vi "Struct Parse Variable Type.vi"(8 "error in":errorcluster, 11 "variant in":variant) -> (0 "error out":errorcluster, 1 "array dims":i16, 2 "data type":T1=enum."Real", 3 "type id":i16)   [LabVIEW 2013, in "GOLPI library.lvlib"]
doc: "Parses 'variable' data type. Obtains data types of the variable, array dimensions count."
uses:
  GOLPI library.lvlib
  Struct Data Types.ctl
panel:
  out "type string":i16[](array[numeric]) format="%04x"
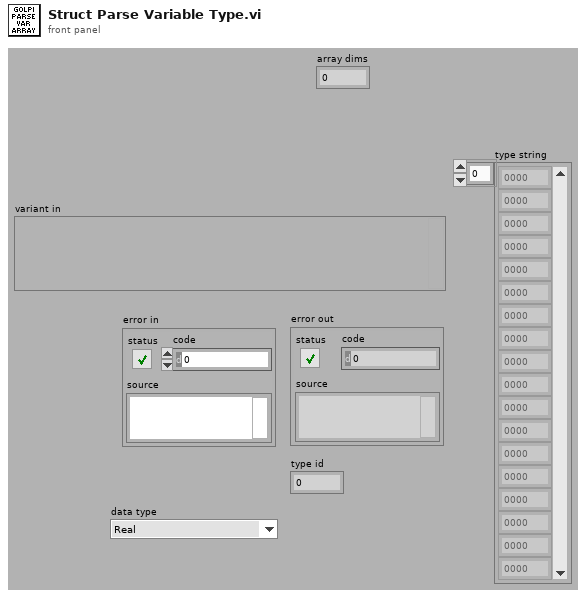
[diagram p1: front panel]
types:
  T1 = typedef "GOLPI library.lvlib/Struct Data Types.ctl" = enum16{"n/a", "Real", "Complex", "String/path", "Cluster", "Bool"}
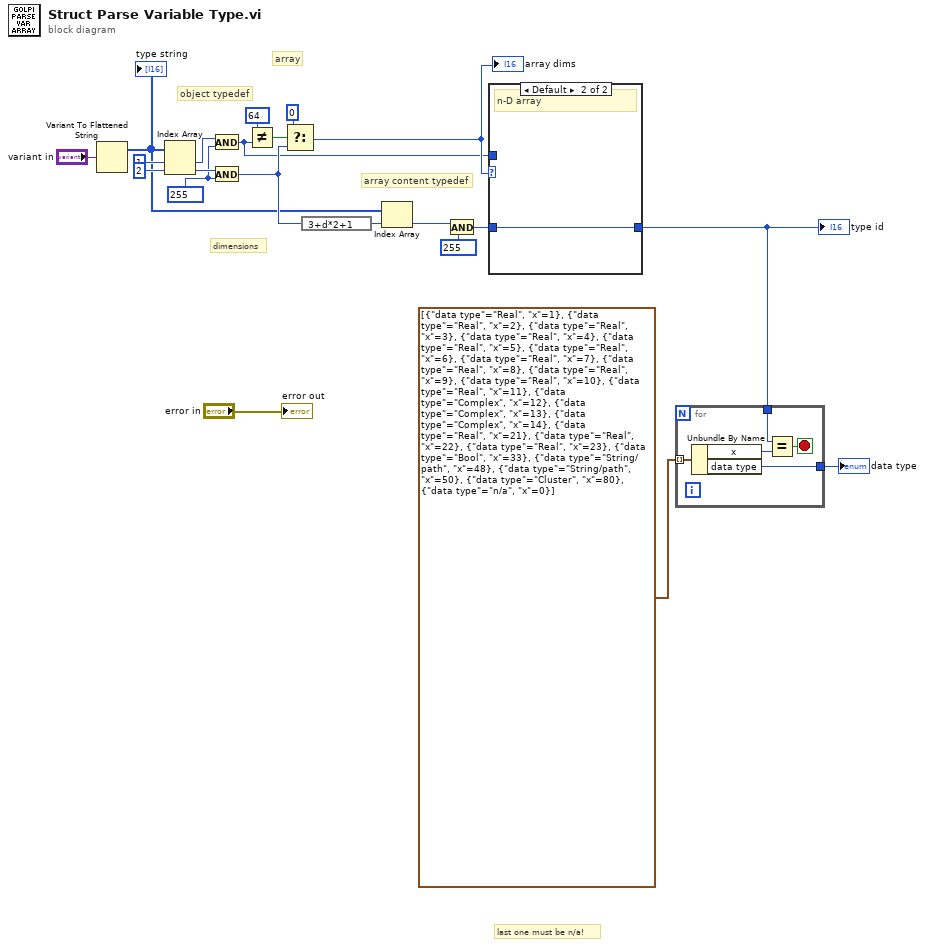
[diagram p0: block diagram]
diagram:
  w13 = i16 255 ("y")
  # "last one must be n/a!"
  # "array content typedef"
  # "dimensions"
  # "array"
  # "object typedef"
  n1 = Variant To Flattened String(Variant="variant in") -> (1:w7:i16[])  [unwired: 1 out]
  "type string" <- w7
  n2 = Index Array(array=w7, index #1=1 ("index"), index #2=2 ("index")) -> (element #1=w14:i16, element #2=w19:i16)
  n3 = And(x=w14, y=w13) -> (x .and. y?=w4:i16)
  n4 = And(x=w19, y=w13) -> (x .and. y?=w8:i16)
  n5 = Not Equal?(x=i16 64, y=w4) -> (x != y?=w11:bool)
  n6 = Select(t=i16 0, s=w11, f=w8) -> (s? t:f=w10:i16)
  "array dims" <- w10
  n7 = expression code="3+d*2+1"(w8) -> (w6:i16)
  n8 = Index Array(array=w7, index=w6) -> (element=w5:i16)
  n9 = And(x=w5, y=i16 255) -> (x .and. y?=w17:i16)
  n10 = case shown="Default" w10 {
    tunnel: w17 -> [_ w23]
    tunnel: [w22 w23] -> w2
    tunnel: w4 -> [w22 _]
    frame 0 {
      # "scalar"
    }
    frame Default {
      # "n-D array"
    }
  }
  "type id" <- w2
  n11 = for {
    tunnel: cluster{"data type":T1, "x":i16}[] [{"data type"=enum."Real", "x"=1}, {"data type"=enum."Real", "x"=2}, {"data type"=enum."Real", "x"=3}, {"data type"=enum."Real", "x"=4}, {"data type"=enum."Real", "x"=5}, {"data type"=enum."Real", "x"=6}, {"data type"=enum."Real", "x"=7}, {"data type"=enum."Real", "x"=8}, {"data type"=enum."Real", "x"=9}, {"data type"=enum."Real", "x"=10}, {"data type"=enum."Real", "x"=11}, {"data type"=enum."Complex", "x"=12}, {"data type"=enum."Complex", "x"=13}, {"data type"=enum."Complex", "x"=14}, {"data type"=enum."Real", "x"=21}, {"data type"=enum."Real", "x"=22}, {"data type"=enum."Real", "x"=23}, {"data type"=enum."Bool", "x"=33}, {"data type"=enum."String/path", "x"=48}, {"data type"=enum."String/path", "x"=50}, {"data type"=enum."Cluster", "x"=80}, {"data type"=enum."n/a", "x"=0}] -> [w28] mode=indexing
    tunnel: w2 -> [w26]
    tunnel: [w25] -> w1
    stop <- w24 stop-if-true
    n12 = Unbundle By Name(w28) -> ("x"=w27:i16, "data type"=w25:T1)
    n13 = Equal?(x=w26, y=w27) -> (x = y?=w24:bool)
  }
  "data type" <- w1
  "error out" <- "error in"
